vi "Read GoogleAPI URI.vi"(8 "error in (no error)":errorcluster, 11 "Oauth2.Google in":refnum<class "Oauth2.Google.lvclass">) -> (0 "error out":errorcluster, 2 "Token Server URI":string, 3 "Oauth2.Google out":refnum<class "Oauth2.Google.lvclass">)   [LabVIEW 2020, in "Oauth2.Google.lvclass"]
uses:
  Oauth2.Google.lvclass
  Oauth2.Google.lvclass/Oauth2.Google.ctl
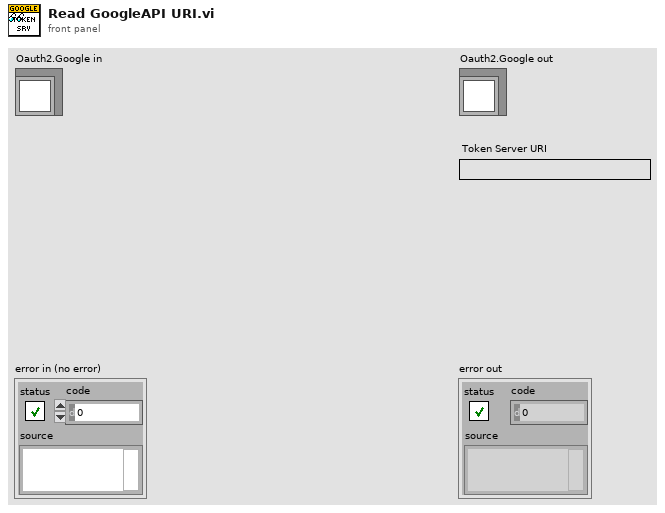
[diagram p1: front panel]
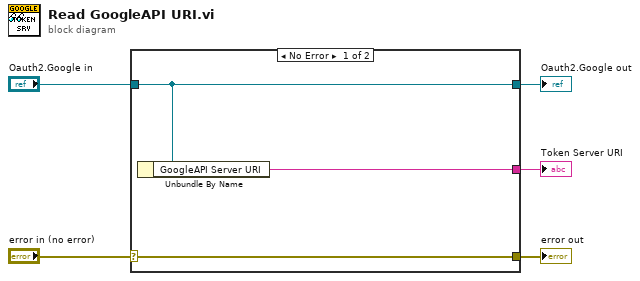
[diagram p0: block diagram]
diagram:
  n1 = case shown="No Error" "error in (no error)" {
    selector: "error in (no error)" -> [w8 w9]
    tunnel: [w8 w9] -> w4
    tunnel: [w7 w10] -> w2
    tunnel: "Oauth2.Google in" -> [w7 w10]
    tunnel: [w6 _] -> w1
    frame No Error {
      n2 = Unbundle By Name(w7) -> ("GoogleAPI Server URI"=w6:string)
    }
    frame Error {
    }
  }
  "error out" <- w4
  "Oauth2.Google out" <- w2
  "Token Server URI" <- w1
